vi "Main.vi"() -> ()   [LabVIEW 2020]
uses:
  <vilib>/IlluminatedG/IG HTTP Server/HTTP Server/Server/Server.lvclass
  <vilib>/IlluminatedG/IG HTTP Server/HTTP Server/StandardFileServe/StandardFileServe.lvclass
  GodotHeaders/GodotHeaders.lvclass
  <vilib>/IlluminatedG/IG WebSocket Stream/Stream-Websocket/Websocket Server/Websocket Server.lvclass
  <vilib>/IlluminatedG/lv-stream/stream/Stream.lvclass
  <vilib>/IlluminatedG/lv-stream/Endpoint/Endpoint.lvclass
  <vilib>/IlluminatedG/IG WebSocket Stream/Stream-Websocket/WebsocketStream/WebsocketStream.lvclass
  <vilib>/IlluminatedG/IG WebSocket Stream/Stream-Websocket/Websocket Client/Websocket Client.lvclass
  C:/Program Files (x86)/National Instruments/LabVIEW 2020/vi.lib/IlluminatedG/lv-stream/stream/Stream.lvclass
  C:/Program Files (x86)/National Instruments/LabVIEW 2020/vi.lib/IlluminatedG/IG WebSocket Stream/Stream-Websocket/WebsocketStream/WebsocketStream.lvclass
  C:/Program Files (x86)/National Instruments/LabVIEW 2020/vi.lib/IlluminatedG/IG HTTP Server/HTTP Server/Controller/Controller.lvclass
  C:/Program Files (x86)/National Instruments/LabVIEW 2020/vi.lib/IlluminatedG/IG HTTP Server/HTTP Server/Handler/Handler.lvclass
  C:/Program Files (x86)/National Instruments/LabVIEW 2020/vi.lib/IlluminatedG/IG HTTP Server/HTTP Server/StandardFileServe/StandardFileServe.lvclass
  C:/Program Files (x86)/National Instruments/LabVIEW 2020/vi.lib/IlluminatedG/IG HTTP Server/HTTP Server/Response Handler/Response Handler.lvclass
  C:/dev/lv20CE/GodotWebTest/GodotHeaders/GodotHeaders.lvclass
  C:/Program Files (x86)/National Instruments/LabVIEW 2020/vi.lib/IlluminatedG/lv-stream/Endpoint/Endpoint.lvclass
  C:/Program Files (x86)/National Instruments/LabVIEW 2020/vi.lib/IlluminatedG/IG WebSocket Stream/Stream-Websocket/Websocket Server/Websocket Server.lvclass
  <vilib>/sklein/WebView2/Webview2 Control/WebView2 Control.xctl
panel:
  out "P X":dbl
  out "P Y":dbl
  out "T X":dbl
  out "T Y":dbl
  out "VY":dbl
  out "VX":dbl
  in  "Skip Page":bool=TRUE
  in  "Throttle":dbl(slide) scale=0.0..1.0
  in  "Thrust Angle":dbl(knob) scale=15.0..-15.0
  out "View":string(xcontrol)
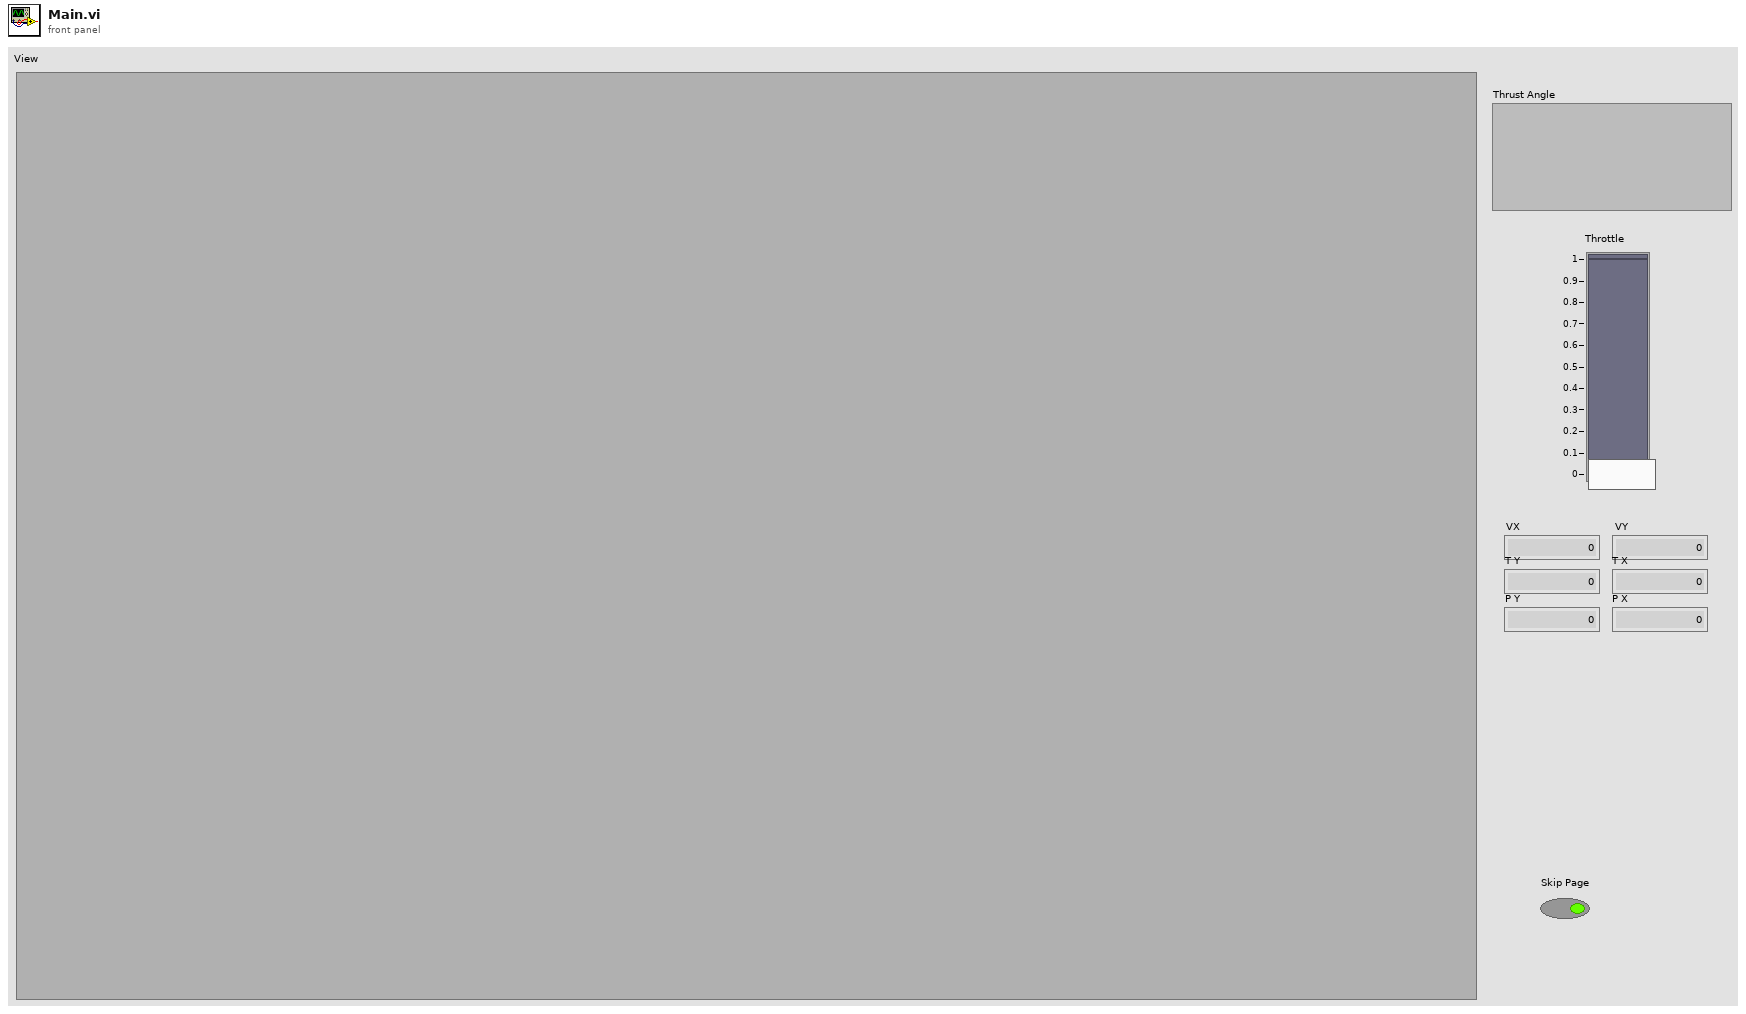
[diagram p1: front panel]
types:
  T1 = cluster{"V.x":dbl, "V.y":dbl, "t.x":dbl, "t.y":dbl, "p.x":dbl, "p.y":dbl}
  T2 = enum16{"big-endian, network order", "native, host order", "little-endian"}
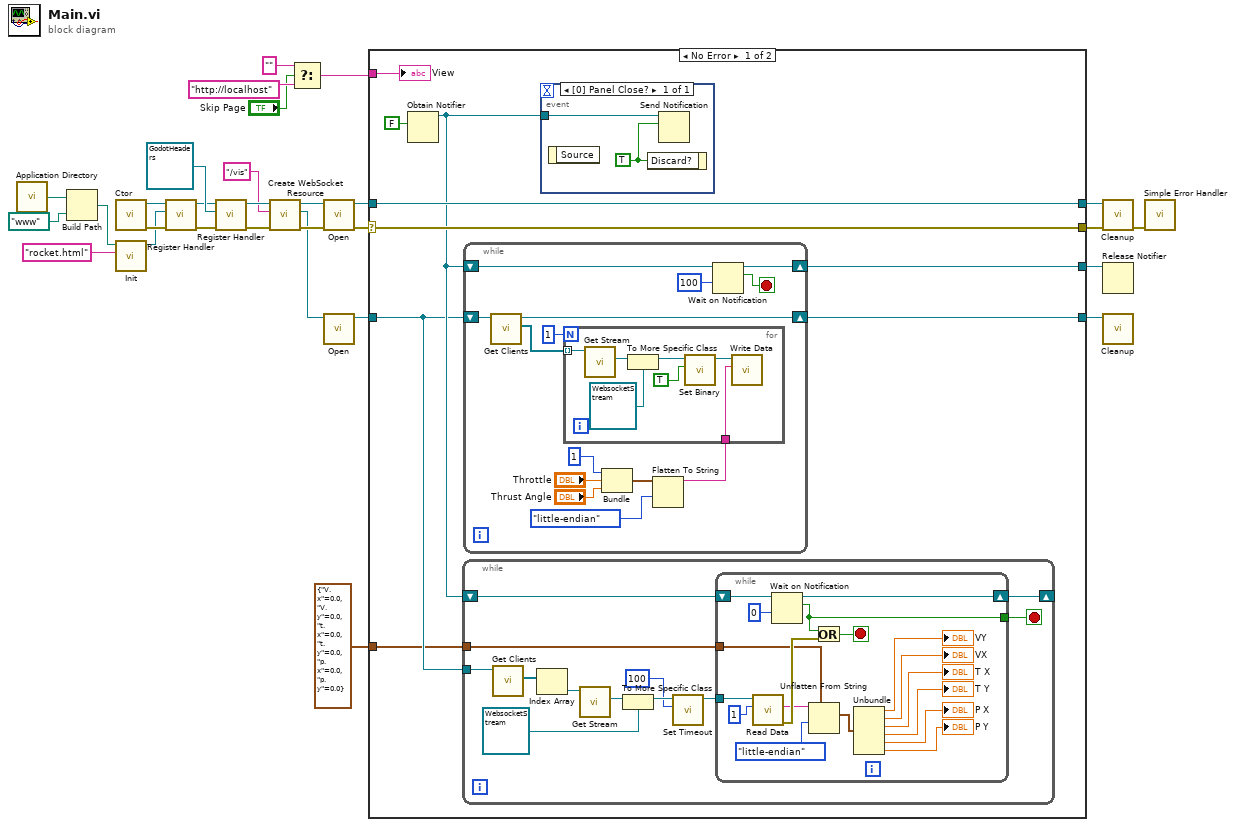
[diagram p0: block diagram]
diagram:
  n1 = call <vilib>:"Application Directory.vi"() -> ("Application Directory"=w3:path)
  n2 = Build Path(base path=w3, name or relative path=path "www") -> (appended path=w1:path)
  n3 = call <vilib>:"Ctor.vi"() -> ("error out"=w28:errorcluster, "Server out"=w29:refnum<class "Server.lvclass">)  [unwired: 10 in]
  n4 = call <vilib>:"Init.vi"("Default Index File (index.html)"="rocket.html", "Public Root"=w1) -> ("StandardFileServe out"=w26:refnum<class "StandardFileServe.lvclass">)  [unwired: 8 in, 1 out]
  n5 = call <vilib>:"Register Handler.vi"("error in (no error)"=w28, "Handler"=w26, "Server in"=w29) -> ("error out"=w18:errorcluster, "Server out"=w19:refnum<class "Server.lvclass">)  [unwired: 7 in]
  n6 = call <vilib>:"Register Handler.vi"("error in (no error)"=w18, "Handler"=refnum<class "GodotHeaders.lvclass"> refnum ("GodotHeaders.lvclass"), "Server in"=w19) -> ("error out"=w15:errorcluster, "Server out"=w17:refnum<class "Server.lvclass">)  [unwired: 7 in]
  n7 = call <vilib>:"Create WebSocket Resource.vi"("error in (no error)"=w15, "Path"="/vis", "Server in"=w17) -> ("error out"=w13:errorcluster, "WS Server"=w6:refnum<class "Websocket Server.lvclass">, "Server out"=w14:refnum<class "Server.lvclass">)  [unwired: 6 in]
  n8 = Select(t="", s="Skip Page", f="http://localhost" ("WebView2 Control")) -> (s? t:f=w9:string)
  n9 = call <vilib>:"Open.vi"("error in (no error)"=w13, "Server in"=w14) -> ("error out"=w25:errorcluster, "Server out"=w24:refnum<class "Server.lvclass">)  [unwired: 8 in]
  n10 = call <vilib>:"Open.vi"("Endpoint in"=w6) -> ("Endpoint out"=w8:refnum<class "Websocket Server.lvclass">)  [unwired: 9 in, 1 out]
  n11 = case shown="No Error" w25 {
    selector: w25 -> [w37 w93]
    tunnel: w24 -> [w38 w94]
    tunnel: [w38 w94] -> w23
    tunnel: [w37 w93] -> w22
    tunnel: w8 -> [w31 w92]
    tunnel: w9 -> [w35 _]
    tunnel: [w34 w92] -> w7
    tunnel: [w32 _] -> w5
    tunnel: T1 {"V.x"=0.0, "V.y"=0.0, "t.x"=0.0, "t.y"=0.0, "p.x"=0.0, "p.y"=0.0} -> [w30 _]
    frame No Error {
      n12 = Obtain Notifier(notification data type=FALSE) -> (notifier out=w33:refnum<notifier>)  [unwired: 3 in, 2 out]
      n13 = while {
        shift-right: [w49] -> _
        shift-left: w33 -> [w50]
        tunnel: w31 -> [w46]
        tunnel: w30 -> [w39]
        stop <- w48 stop-if-true
        n14 = call <vilib>:"Get Clients.vi"("Websocket Server in"=w46) -> ("Clients"=w45:refnum<class "Websocket Client.lvclass">[])  [unwired: 8 in, 2 out]
        n15 = Index Array(array=w45) -> (element=w44:refnum<class "Websocket Client.lvclass">)  [unwired: 1 in]
        n16 = call-dynamic "Get Stream.vi"("Websocket Client in"=w44) -> ("Stream"=w47:refnum<class "Stream.lvclass">)  [unwired: 8 in, 2 out]
        n17 = To More Specific Class(target class=refnum<class "WebsocketStream.lvclass"> refnum ("WebsocketStream in"), reference=w47) -> (specific class reference=w42:refnum<class "WebsocketStream.lvclass">)  [unwired: 1 in, 1 out]
        n18 = call <vilib>:"Set Timeout.vi"("Timeout ms"=100, "WebsocketStream in"=w42) -> ("WebsocketStream out"=w40:refnum<class "WebsocketStream.lvclass">)  [unwired: 8 in, 1 out]
        n19 = while {
          tunnel: [w64] -> w48
          shift-right: [w65] -> w49
          shift-left: w50 -> [w66]
          tunnel: w40 -> [w63]
          tunnel: w39 -> [w55]
          stop <- w56 stop-if-true
          n20 = call <vilib>:"Read Data.vi"("Count"=1, "Stream in"=w63) -> ("error out"=w68:errorcluster, "Data"=w61:string)  [unwired: 7 in, 1 out]
          n21 = Wait on Notification(notifier=w66, timeout in ms (-1)=0) -> (notifier out=w65:refnum<notifier>, notification=w64:bool)  [unwired: 2 in, 2 out]
          n22 = Unflatten From String(type=w55, binary string=w61, byte order (0:big-endian, network order)=T2."little-endian") -> (value=w59:T1)  [unwired: 2 in, 2 out]
          n23 = Or(x=w64, y=w68) -> (x .or. y?=w56:bool)
          n24 = Unbundle(w59) -> ("V.x"=→"VY":dbl, "V.y"=→"VX":dbl, "t.x"=→"T X":dbl, "t.y"=→"T Y":dbl, "p.x"=→"P X":dbl, "p.y"=→"P Y":dbl)
        }
      }
      n25 = while {
        shift-right: [w76] -> w34
        shift-left: w31 -> [w78]
        shift-right: [w72] -> w32
        shift-left: w33 -> [w74]
        stop <- w73 stop-if-true
        n26 = call <vilib>:"Get Clients.vi"("Websocket Server in"=w78) -> ("Clients"=w69:refnum<class "Websocket Client.lvclass">[], "Websocket Server out"=w76:refnum<class "Websocket Server.lvclass">)  [unwired: 8 in, 1 out]
        n27 = Bundle(u8 1, "Throttle"="Throttle", "Thrust Angle"="Thrust Angle") -> (w79:cluster{u8, "Throttle":dbl, "Thrust Angle":dbl})  [unwired: 1 in]
        n28 = Flatten To String(anything=w79, byte order (0:big-endian, network order)=T2."little-endian") -> (data string=w77:string)  [unwired: 2 in, 2 out]
        n29 = for {
          N: 1 -> [_]
          tunnel: w77 -> [w89]
          tunnel: w69 -> [w83] mode=indexing
          n30 = call-dynamic "Get Stream.vi"("Websocket Client in"=w83) -> ("Stream"=w86:refnum<class "Stream.lvclass">)  [unwired: 8 in, 2 out]
          n31 = To More Specific Class(target class=refnum<class "WebsocketStream.lvclass"> refnum ("WebsocketStream in"), reference=w86) -> (specific class reference=w84:refnum<class "WebsocketStream.lvclass">)  [unwired: 1 in, 1 out]
          n32 = call <vilib>:"Set Binary.vi"("Binary"=TRUE, "WebsocketStream in"=w84) -> ("WebsocketStream out"=w87:refnum<class "WebsocketStream.lvclass">)  [unwired: 8 in, 1 out]
          n33 = call <vilib>:"Write Data.vi"("Data"=w89, "Stream in"=w87) -> ()  [unwired: 8 in, 2 out]
        }
        n34 = Wait on Notification(notifier=w74, timeout in ms (-1)=100) -> (notifier out=w72:refnum<notifier>, notification=w73:bool)  [unwired: 2 in, 2 out]
      }
      n35 = event shown="[0] Panel Close?" {
        selector: _ -> [_]
        dyn-events: _ -> [_]
        timeout: _ -> [_]
        tunnel: w33 -> [w90]
        event Panel Close? {
          w91 = TRUE ("Discard?")
          n36 = event-data() -> ()  [unwired: 1 in, 1 out]
          n37 = event-data("Discard?"=w91) -> ()  [unwired: 1 in, 1 out]
          n38 = Send Notification(notification=w91, notifier=w90) -> ()  [unwired: 1 in, 2 out]
        }
      }
      "View" <- w35
    }
    frame Error {
    }
  }
  n39 = call <vilib>:"Cleanup.vi"("error in (no error)"=w22, "Server in"=w23) -> ("error out"=w21:errorcluster)  [unwired: 9 in]
  n40 = Release Notifier(notifier=w5) -> ()  [unwired: 2 in, 3 out]
  n41 = call-dynamic <vilib>:"Cleanup.vi"("Websocket Server in"=w7) -> ()  [unwired: 10 in, 1 out]
  n42 = call <vilib>:"Simple Error Handler.vi"("error in (no error)"=w21) -> ()  [unwired: 4 in, 5 out]
